vi "nanomsg_sub.vi"() -> ()   [LabVIEW 2014]
uses:
  lvnanomsg/nanomsg_context.lvclass
  lvnanomsg/nanomsg_socket.lvclass
panel:
  in  "ports":i32[](array[numeric])=[5555, 5556, 5557]
  out "messages":string[](array[string])
  # "Nanomsg subscriber VI"
  # "Subscribe to all messages published to specified ports"
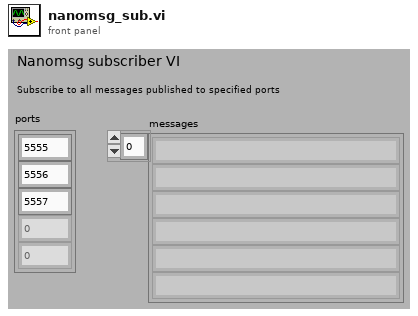
[diagram p1: front panel]
types:
  T1 = enum16{"NN_SUB_XXX", "NN_SUB_SUBSCRIBE", "NN_SUB_UNSUBSCRIBE"}
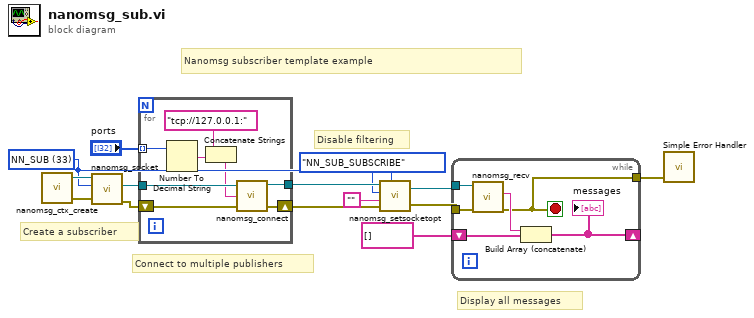
[diagram p0: block diagram]
diagram:
  w1 = 33 items=["NN_WS"=-4, "NN_TCP"=-3, "NN_IPC"=-2, "NN_INPROC"=-1, "NN_SOL_SOCKET"=0, "NN_PAIR"=16, "NN_PUB"=32, "NN_SUB"=33, "NN_REQ"=48, "NN_REP"=49, "NN_PUSH"=80, "NN_PULL"=81, "NN_SURVEYOR"=98, "NN_RESPONDENT"=99, "NN_BUS"=112] ("socket type")
  # "Nanomsg subscriber template example"
  # "Display all messages"
  # "Create a subscriber"
  # "Disable filtering"
  # "Connect to multiple publishers"
  n1 = call "nanomsg_ctx_create.vi"() -> ("error out"=w13:errorcluster, "context out"=w14:refnum<class "nanomsg_context.lvclass">)  [unwired: 4 in]
  n2 = call "nanomsg_socket.vi"("error in"=w13, "socket type"=w1, "context in"=w14) -> ("error out"=w12:errorcluster, "socket out"=w2:refnum<class "nanomsg_socket.lvclass">)  [unwired: 2 in, 1 out]
  n3 = for {
    tunnel: w2 -> [w22]
    tunnel: [w19] -> w11
    tunnel: "ports" -> [w15] mode=indexing
    shift-right: [w18] -> w10
    shift-left: w12 -> [w21]
    n4 = Number To Decimal String(number=w15) -> (decimal integer string=w16:string)  [unwired: 1 in]
    n5 = Concatenate Strings("tcp://127.0.0.1:" ("endpoint"), w16) -> (w17:string)
    n6 = call "nanomsg_connect.vi"("error in"=w21, "endpoint"=w17, "socket in"=w22) -> ("error out"=w18:errorcluster, "socket out"=w19:refnum<class "nanomsg_socket.lvclass">)  [unwired: 1 in]
  }
  n7 = call "nanomsg_setsocketopt.vi"("socket in"=w11, "option"=T1."NN_SUB_SUBSCRIBE", "value"="", "error in"=w10, "level"=w1) -> ("socket out"=w8:refnum<class "nanomsg_socket.lvclass">, "error out"=w9:errorcluster)
  n8 = while {
    tunnel: w8 -> [w28]
    tunnel: w9 -> [w27]
    shift-right: [w24] -> _
    shift-left: string[] [] -> [w25]
    tunnel: [w23] -> w3
    stop <- w23 stop-if-true
    n9 = call "nanomsg_recv.vi"("error in"=w27, "socket in"=w28) -> ("error out"=w23:errorcluster, "data"=w26:string)  [unwired: 3 in, 3 out]
    n10 = Build Array (concatenate)(w26, w25) -> (w24:string[])
    "messages" <- w24
  }
  n11 = call <vilib>:"Simple Error Handler.vi"("error in (no error)"=w3) -> ()  [unwired: 4 in, 5 out]
